vi "Do.vi"(8 "error in (no error)":errorcluster, 10 "Actor in":refnum<class "Actor.lvclass">, 11 "Write Selected DTRows Msg":refnum<class "Write Selected DTRows Msg.lvclass">) -> (0 "error out":errorcluster, 2 "Actor out":refnum<class "Actor.lvclass">)   [LabVIEW 2016, in "Controller UI.lvlib" / "Write Selected DTRows Msg.lvclass"]
doc: "This VI delivers the message to the actor by calling the appropriate method(s) on the actor."
uses:
  <userlib>/Common Components/Controller UI Messages/Write Selected DTRows Msg/Write Selected DTRows Msg.lvclass
  <vilib>/ActorFramework/Actor/Actor.lvclass
  <userlib>/Common Components/Controller UI/Controller UI.lvclass
  C:/Program Files (x86)/National Instruments/LabVIEW 2016/vi.lib/ActorFramework/Actor/Actor.lvclass
  <userlib>/Common Components/Controller UI Messages/Write Selected DTRows Msg/Write Selected DTRows Msg.lvclass/Write Selected DTRows Msg.ctl
  <userlib>/Common Components/Controller UI/Controller UI.lvclass/Controller UI.ctl
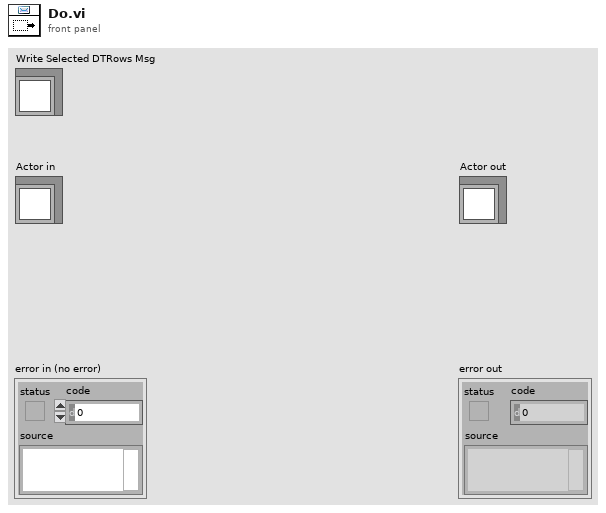
[diagram p1: front panel]
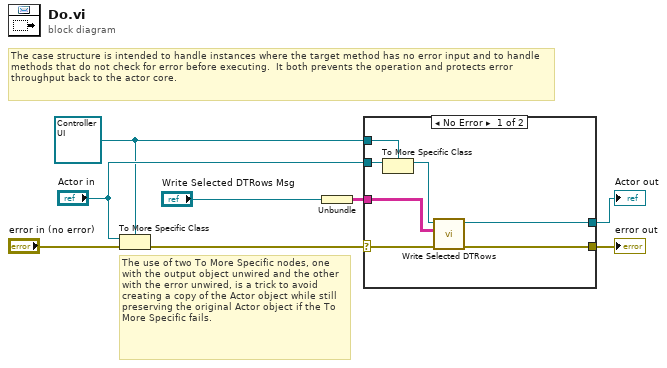
[diagram p0: block diagram]
diagram:
  w2 = refnum<class "Controller UI.lvclass"> refnum ("Actor in")
  # "The use of two To More Specific nodes, one with the output object unwired and the other with the error unwired, is a trick to avoid creating a copy of the Actor object while still preserving the original Actor object if the To More Specific fails."
  # "The case structure is intended to handle instances where the target method has no error input and to handle methods that do not check for error before executing.  It both prevents the operation and protects error throughput back to the actor core."
  n1 = To More Specific Class(target class=w2, reference="Actor in", error in="error in (no error)") -> (error out=w6:errorcluster)  [unwired: 1 out]
  n2 = Unbundle("Write Selected DTRows Msg") -> (w1:string[][])
  n3 = case shown="No Error" w6 {
    selector: w6 -> [w13 w17]
    tunnel: [w15 w17] -> w5
    tunnel: [w14 w16] -> w4
    tunnel: "Actor in" -> [w12 w16]
    tunnel: w2 -> [w11 _]
    tunnel: w1 -> [w9 _]
    frame No Error {
      n4 = To More Specific Class(target class=w11, reference=w12) -> (specific class reference=w10:refnum<class "Controller UI.lvclass">)  [unwired: 1 in, 1 out]
      n5 = call <userlib>:"Write Selected DTRows.vi"("error in (no error)"=w13, "Selected DTRows"=w9, "Controller UI in"=w10) -> ("error out"=w15:errorcluster, "Controller UI out"=w14:refnum<class "Controller UI.lvclass">)  [unwired: 7 in]
    }
    frame Error {
      # "If type check fails, pass the original object out again."
    }
  }
  "error out" <- w5
  "Actor out" <- w4
